vi "fmt_timestampToExcel.vi"(11 "timestamp":timestamp) -> (3 "Excel timestamp":dbl format="%#_30g")   [LabVIEW 2020, in "NI_ExcelFile.lvlib"]
uses:
  <vilib>/express/express shared/NI_ExcelFile/NI_ExcelFile.lvlib
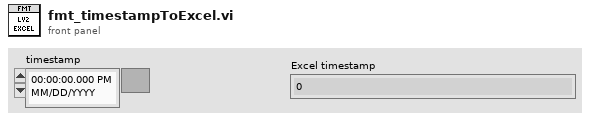
[diagram p1: front panel]
types:
  T1 = typedef "LVDateTimeRec.ctl" = cluster{"fractional second":dbl, "second":i32, "minute":i32, "hour":i32, "day of month":i32, "month":i32, "year":i32, "day of week":i32, "day of year":i32, "DST":i32}
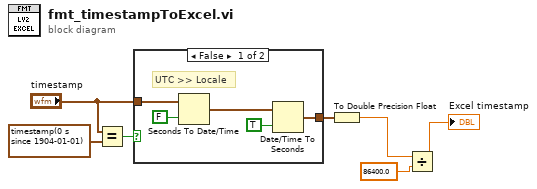
[diagram p0: block diagram]
diagram:
  n1 = Equal?(x="timestamp", y=timestamp(0 s since 1904-01-01)) -> (x = y?=w5:bool)
  n2 = case shown="False" w5 {
    tunnel: "timestamp" -> [w12 w13]
    tunnel: [w11 w13] -> w7
    frame False {
      # "UTC >> Locale"
      n3 = Seconds To Date/Time(time stamp (now)=w12, to UTC (F)=FALSE) -> (date time rec=w8:T1)
      n4 = Date/Time To Seconds(1:TRUE ("is UTC (F)"), 2:w8) -> (0:w11:timestamp)
    }
    frame True {
    }
  }
  n5 = To Double Precision Float(number=w7) -> (double precision float=w2:dbl)
  n6 = Divide(x=w2, y=86400.0) -> (x/y=→"Excel timestamp":dbl)
